vi "Loop_HW_Wheel.vi"() -> ()   [LabVIEW 2017, in "Shooter.lvlib"]
uses:
  Shooter.lvlib
  _SHARE ALL/Global Share All/Global_STOP.vi
  Global_SM_Data Out.vi
  Global_HW Status.vi
  Globals/Global_HW_Address_Assignments.vi
  <vilib>/Rock Robotics/WPI/MotorControl/WPI_MotorControlType.ctl
  <vilib>/Rock Robotics/SystemInterfaces/DIO/FPGA_DIOPWMChannel.ctl
  <vilib>/Rock Robotics/WPI/PWM/WPI_PWMDeadband.ctl
  <vilib>/Rock Robotics/SystemInterfaces/DIO/FPGA_DIOChannel.ctl
  <vilib>/Rock Robotics/WPI/MotorControl/WPI_MotorControlDeviceRef.ctl
  TypeDefs/Cluster_SRX Status With Encoder.ctl
  TypeDefs/Cluster_SRX PID Values.ctl
panel:
  out "Vbus":dbl(graph)
  out "Sensor Values":cluster{"Fly Wheel RPM In":dbl, dbl}(graph)={"Fly Wheel RPM In"=1624.8046875, 0.0}
  in  "Fly Wheel PID":T1={"P"=0.35, "I"=0.0, "D"=0.0, "F"=0.04, "I Zone"=0.0, "Ramp Rate"=0.0}
  out "Wheel Status":T2={"VBus "=0.0, "Module Enabled"=TRUE, "Closed Loop Error"=-11074.0, "Sensor Pos"=16383.998046875, "Sensor Vel"=1624.8046875, "Current"=0.75, "Brake is Enabled"=FALSE, "Encoder Pos"=-67108864.0, "Encoder Vel"=-11209.0, " APin"=FALSE, "B Pin"=TRUE, "Bat Voltage"=12.55, "Profile Slot"=0.0}
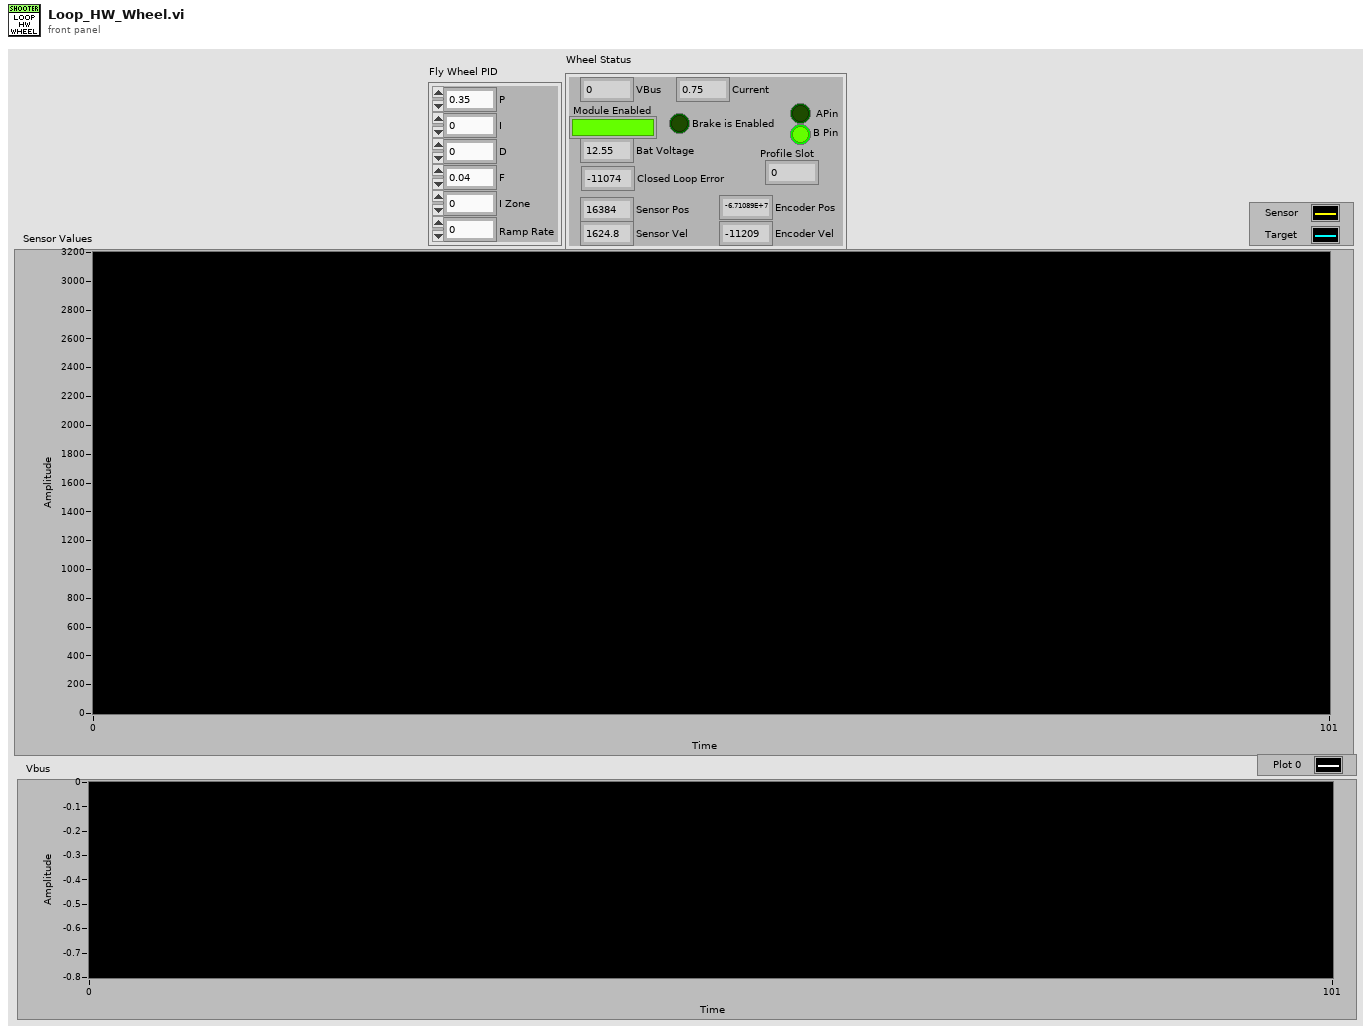
[diagram p1: front panel]
types:
  T1 = typedef "Cluster_SRX PID Values.ctl" = cluster{"P":dbl, "I":dbl, "D":dbl, "F":dbl, "I Zone":dbl, "Ramp Rate":dbl}
  T2 = typedef "Cluster_SRX Status With Encoder.ctl" = cluster{"VBus ":dbl, "Module Enabled":bool, "Closed Loop Error":dbl, "Sensor Pos":dbl, "Sensor Vel":dbl, "Current":dbl, "Brake is Enabled":bool, "Encoder Pos":dbl, "Encoder Vel":dbl, " APin":bool, "B Pin":bool, "Bat Voltage":dbl, "Profile Slot":dbl}
  T3 = typedef "WPI_MotorControlDeviceRef.ctl" = cluster{"DeviceStatus":errorcluster, "Type":T4, "PWM":cluster{"PWM Channel":T5, "DeadBand":T6}, "CAN":cluster{"Device Number":u8, "SetOutput VI Ref":variant, "GetOutput VI Ref":variant, "Enable VI Ref":variant, "Disable VI Ref":variant, "Data":variant}, "Invert":bool, "DIO PWM":cluster{"PWM \"Enable\" Channel":T5, "DIOChannel":T7, "PWM Rate":dbl}}
  T4 = typedef "WPI_MotorControlType.ctl" = enum16{"PWM", "CAN", "DIO PWM"}
  T5 = typedef "FPGA_DIOPWMChannel.ctl" = enum8{"PWM 0", "PWM 1", "PWM 2", "PWM 3", "PWM 4", "PWM 5", "PWM 6", "PWM 7", "PWM 8", "PWM 9", "PWM MXP 0", "PWM MXP 1", "PWM MXP 2", "PWM MXP 3", "PWM MXP 4", "PWM MXP 5", "PWM MXP 6", "PWM MXP 7", "PWM MXP 8", "PWM MXP 9", "Invalid"}
  T6 = typedef "WPI_PWMDeadband.ctl" = cluster{"Name":string, "maxPositivePwm":i32, "minPositivePwm":i32, "centerPwm":i32, "maxNegativePwm":i32, "minNegativePwm":i32, "angularRange":u16}
  T7 = typedef "FPGA_DIOChannel.ctl" = enum8{"DIO 0", "DIO 1", "DIO 2", "DIO 3", "DIO 4", "DIO 5", "DIO 6", "DIO 7", "DIO 8", "DIO 9", "DIO MXP 0", "DIO MXP 1", "DIO MXP 2", "DIO MXP 3", "DIO MXP 4", "DIO MXP 5", "DIO MXP 6", "DIO MXP 7", "DIO MXP 8", "DIO MXP 9", "DIO MXP 10", "DIO MXP 11", "DIO MXP 12", "DIO MXP 13", "DIO MXP 14", "DIO MXP 15", "SPI Port CS1", "SPI Port CS2", "SPI Port CS3", "SPI Port MISO", "SPI Port MOSI", "Invalid"}
  T8 = typedef "Shooter.lvlib/Cluster_SM to HW Wheel Data.ctl" = cluster{"Use Encoder":bool, "VBus":dbl, "RPM":dbl}
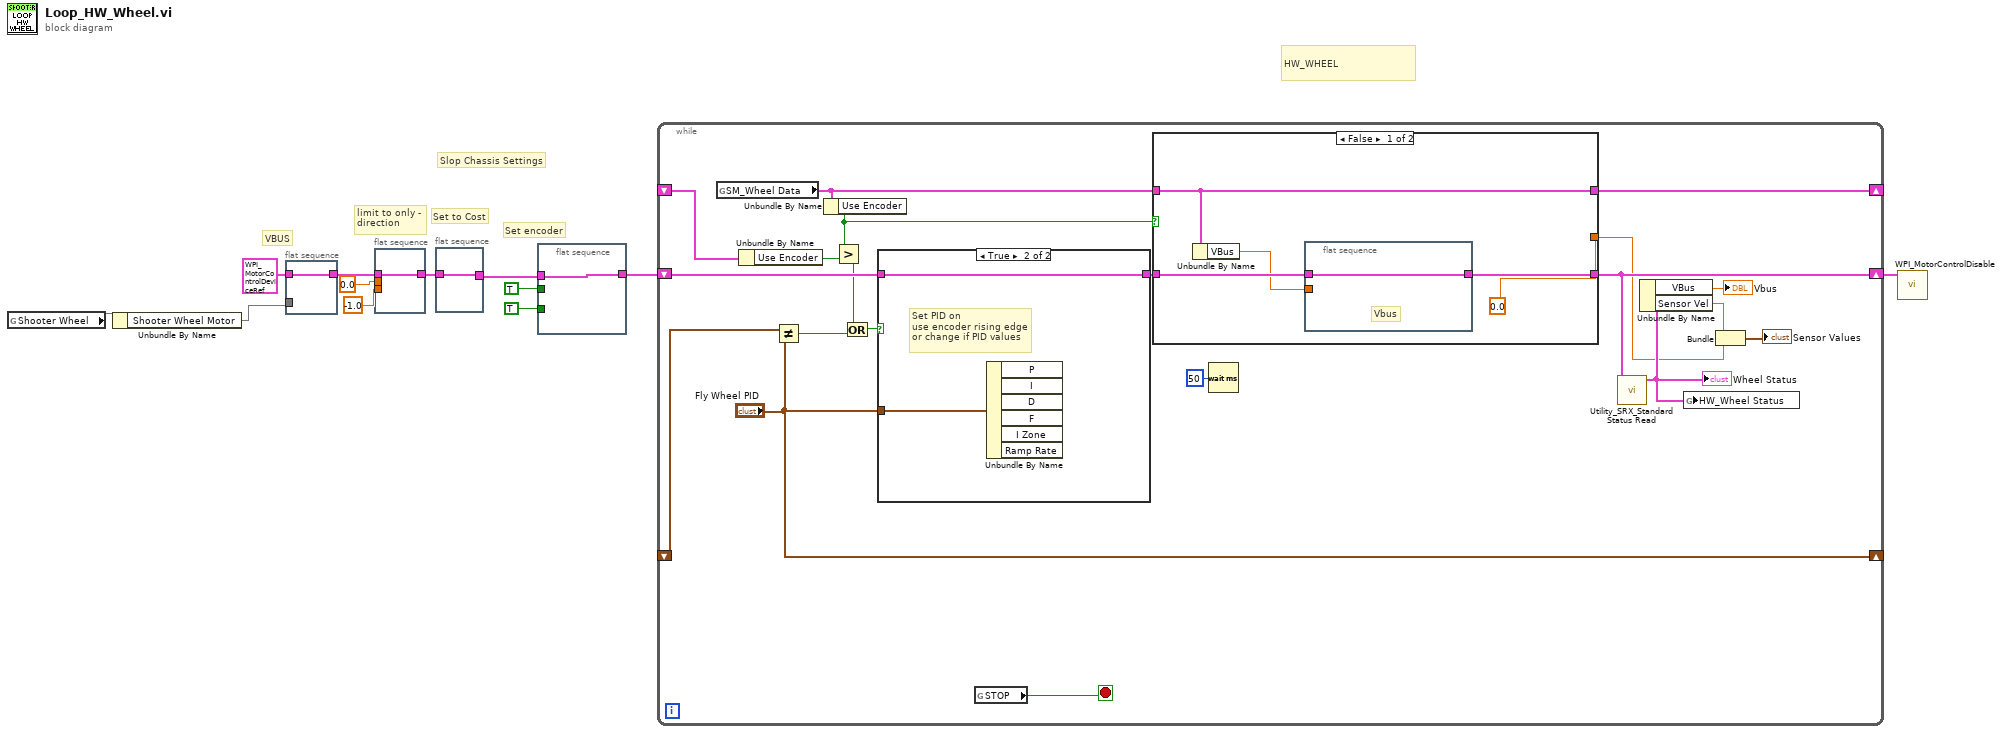
[diagram p0: block diagram]
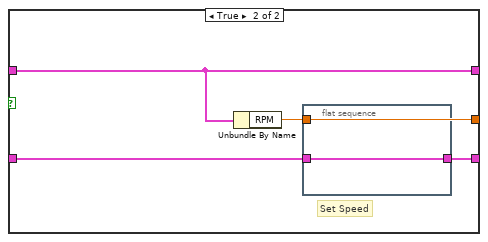
[diagram p3: hidden frame]
diagram:
  # "Set encoder"
  # "limit to only -\ndirection"
  # "Set to Cost"
  # "VBUS"
  # "HW_WHEEL"
  # "Slop Chassis Settings"
  n1 = global read "Global_HW_Address_Assignments.vi" "Shooter Wheel"() -> (w4)
  n2 = Unbundle By Name(w4) -> ("Shooter Wheel Motor"=w3)
  n3 = flat-sequence {
    tunnel: [w13] -> w8
    tunnel: w3 -> [_]
    tunnel: T3 {"DeviceStatus"={"status"=FALSE, "code"=0, "source"=""}, "Type"=enum."PWM", "PWM"={"PWM Channel"=enum."Invalid", "DeadBand"={"Name"="", "maxPositivePwm"=0, "minPositivePwm"=0, "centerPwm"=0, "maxNegativePwm"=0, "minNegativePwm"=0, "angularRange"=0}}, "CAN"={"Device Number"=0, "SetOutput VI Ref"=variant, "GetOutput VI Ref"=variant, "Enable VI Ref"=variant, "Disable VI Ref"=variant, "Data"=variant}, "Invert"=FALSE, "DIO PWM"={"PWM \"Enable\" Channel"=enum."Invalid", "DIOChannel"=enum."Invalid", "PWM Rate"=0.0}} ("CAN Talon SRX Ref") -> [w13]
    frame #0 {
    }
  }
  n4 = flat-sequence {
    tunnel: 0.0 ("Forward Peak Output") -> [_]
    tunnel: -1.0 ("Reverse Peak Output") -> [_]
    tunnel: w8 -> [w14]
    tunnel: [w14] -> w7
    frame #0 {
    }
  }
  n5 = flat-sequence {
    tunnel: [w15] -> w1
    tunnel: w7 -> [w15]
    frame #0 {
    }
  }
  n6 = flat-sequence {
    tunnel: TRUE ("Reverse Feedback Sensor") -> [_]
    tunnel: TRUE ("Reverse Closed-Loop Output") -> [_]
    tunnel: [w16] -> w5
    tunnel: w1 -> [w16]
    frame #0 {
    }
  }
  n7 = while {
    shift-right: [w23] -> w12
    shift-left: w5 -> [w34]
    shift-right: ["Fly Wheel PID"] -> _
    shift-left: _ -> [w32]
    shift-right: [w25] -> _
    shift-left: _ -> [w29]
    stop <- w36 stop-if-true
    n8 = global read "Global_SM_Data Out.vi" "SM_Wheel Data"() -> (w24:T8)
    n9 = Unbundle By Name(w29) -> ("Use Encoder"=w27:bool)
    n10 = Not Equal?(x=w32, y="Fly Wheel PID") -> (x != y?=w31:bool)
    n11 = Unbundle By Name(w24) -> ("Use Encoder"=w26:bool)
    n12 = Greater?(x=w26, y=w27) -> (0:w28:bool)
    n13 = Or(x=w28, y=w31) -> (x .or. y?=w30:bool)
    n14 = case shown="True" w30 {
      tunnel: w34 -> [w37 w38]
      tunnel: [w37 w38] -> w33
      tunnel: "Fly Wheel PID" -> [_ w39]
      frame False {
      }
      frame True {
        # "Set PID on\nuse encoder rising edge\nor change if PID values"
        n15 = Unbundle By Name(w39) -> ()  [unwired: 6 out]
      }
    }
    n16 = global read "Global_STOP.vi" "STOP"() -> (w36:bool)
    n17 = case shown="False" w26 {
      tunnel: [w44 w48] -> w23
      tunnel: w33 -> [w43 w49]
      tunnel: w24 -> [w42 w47]
      tunnel: [w42 w47] -> w25
      tunnel: [0.0 ("RPM") w46] -> w18
      frame False {
        n18 = Unbundle By Name(w42) -> ("VBus"=w41:dbl)
        n19 = flat-sequence {
          tunnel: [w45] -> w44
          tunnel: w43 -> [w45]
          tunnel: w41 -> [_]
          frame #0 {
            # "Vbus"
          }
        }
      }
      frame True {
        # "Set Speed"
        n20 = Unbundle By Name(w47) -> ("RPM"=w46:dbl)
        n21 = flat-sequence {
          tunnel: w49 -> [w50]
          tunnel: [w50] -> w48
          tunnel: w46 -> [_]
          frame #0 {
          }
        }
      }
    }
    n22 = Wait (ms)(milliseconds to wait=u32 50) -> ()  [unwired: 1 out]
    n23 = call "Utility_SRX_Standard Status Read.vi"("SingleMotorRef"=w23) -> ("SRX With Encoder Out"=w21:T2)  [unwired: 8 in, 2 out]
    "Wheel Status" <- w21
    n24 = Unbundle By Name(w21) -> ("VBus"=→"Vbus":dbl, "Sensor Vel"=w19:dbl)
    n25 = global write "Global_HW Status.vi" "HW_Wheel Status"(w21) -> ()
    n26 = Bundle("Sensor Vel"=w19, "RPM"=w18) -> (→"Sensor Values":cluster{"Sensor Vel":dbl, "RPM":dbl})  [unwired: 1 in]
  }
  n27 = call <vilib>:"WPI_MotorControlDisable.vi"("MotorControlDevRef"=w12) -> ()  [unwired: 9 in, 2 out]
